vi "Task Monitor Using .NET Objects.vi"() -> ()   [LabVIEW 2023]
doc: "The Task Monitor uses .NET assemblies to monitor basic CPU and system memory usage. It uses the PerformanceCounter class to get the CPU usage and also to determine how much memory is being used. \n\nThe example makes use of the System.Diagnostics.PerformanceCounter class. The PerformanceCounter category names and counterNames were obtained from the Microsoft documentation for the PerformanceCounter class. For more information about the various .NET libraries used in this example, refer to the Microsoft Developers Network at msdn.microsoft.com."
panel:
  out "CPU Usage History":sgl(graph)
  out "Memory Usage History":sgl(graph)
  in  "Stop":bool
  # "Overview: Implements a simple task monitor using .NET objects.\nRequirements: Windows\nInstructions:\n1. Ensure you are logged in to Windows with administrator privileges.\n2. Run the VI.\n3. Observe the system information being monitored using .NET objects.\n4. Click Stop to stop the VI."
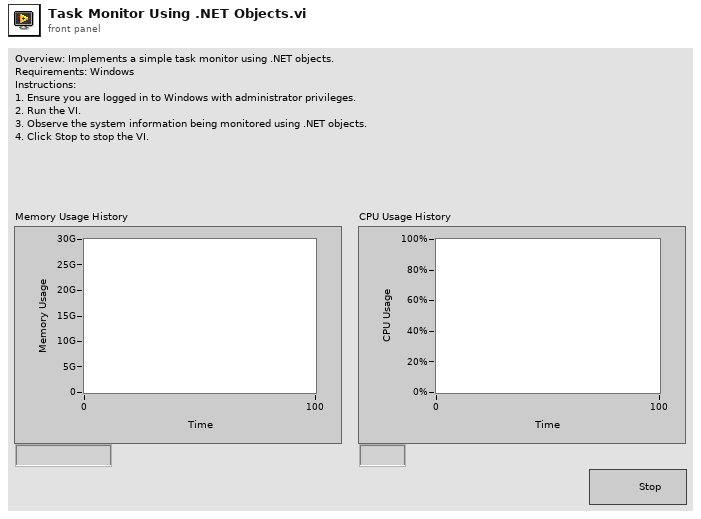
[diagram p1: front panel]
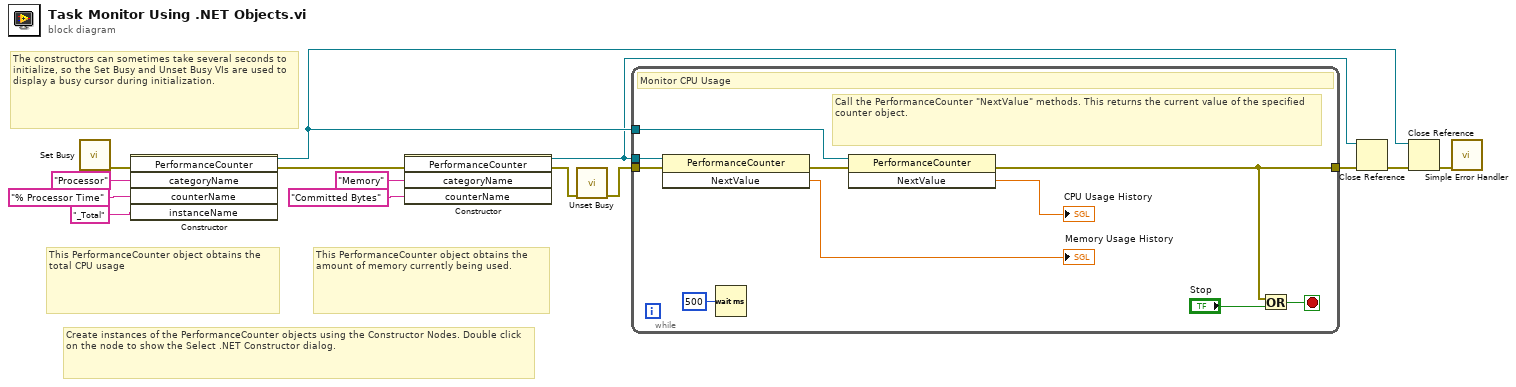
[diagram p0: block diagram]
diagram:
  # "The constructors can sometimes take several seconds to initialize, so the Set Busy and Unset Busy VIs are used to display a busy cursor during initialization."
  # "Create instances of the PerformanceCounter objects using the Constructor Nodes. Double click on the node to show the Select .NET Constructor dialog."
  # "This PerformanceCounter object obtains the amount of memory currently being used."
  # "This PerformanceCounter object obtains the total CPU usage"
  n1 = call <vilib>:"Set Busy.vi"() -> ("error out"=w3:errorcluster)  [unwired: 10 in, 1 out]
  n2 = constructor class="PerformanceCounter"(error in=w3, "categoryName"="Processor", "counterName"="% Processor Time", "instanceName"="_Total") -> (reference out=w5:refnum<k24>, error out=w10:errorcluster)  [unwired: 2 in, 4 out]
  n3 = constructor class="PerformanceCounter"(error in=w10, "categoryName"="Memory", "counterName"="Committed Bytes") -> (reference out=w4:refnum<k24>, error out=w2:errorcluster)  [unwired: 2 in, 3 out]
  n4 = call <vilib>:"Unset Busy.vi"("error in (no error)"=w2) -> ("error out"=w1:errorcluster)  [unwired: 10 in]
  n5 = while {
    tunnel: w5 -> [w21]
    tunnel: w4 -> [w20]
    tunnel: w1 -> [w16]
    tunnel: [w19] -> w9
    stop <- w22 stop-if-true
    # "Call the PerformanceCounter \"NextValue\" methods. This returns the current value of the specified counter object."
    # "Monitor CPU Usage"
    n6 = invoke class="PerformanceCounter" method="NextValue"(reference=w20, error in=w16) -> (error out=w15:errorcluster, "NextValue"=→"Memory Usage History":sgl)  [unwired: 1 in, 1 out]
    n7 = Wait (ms)(milliseconds to wait=u32 500 ("millisecond multiple")) -> ()  [unwired: 1 out]
    n8 = invoke class="PerformanceCounter" method="NextValue"(reference=w21, error in=w15) -> (error out=w19:errorcluster, "NextValue"=→"CPU Usage History":sgl)  [unwired: 1 in, 1 out]
    n9 = Or(x=w19, y="Stop") -> (x .or. y?=w22:bool)
  }
  n10 = Close Reference(reference=w4, error in (no error)=w9) -> (error out=w11:errorcluster)
  n11 = Close Reference(reference=w5, error in (no error)=w11) -> (error out=w12:errorcluster)
  n12 = call <vilib>:"Simple Error Handler.vi"("error in (no error)"=w12) -> ()  [unwired: 1 in, 8 out]
